vi "Tool Q LEIN stroke fb value ovveride.vi"(1 "Retry on err (F)":bool, 5 "stroke value(mm)":dbl, 9 "Serial number(any number(-1))":i16=-1, 11 "error in (no error)":errorcluster) -> (15 "error out":errorcluster)   [LabVIEW 2011]
doc: "-1 = any address:\n-2 = do not update"
uses:
  LEINmaster/Defenitions/LEIN Structure variations.ctl
  Application Structure/Options/Action GFV Settings.ctl
panel:
  # "-1 = any address:\n-2 =  do not update"
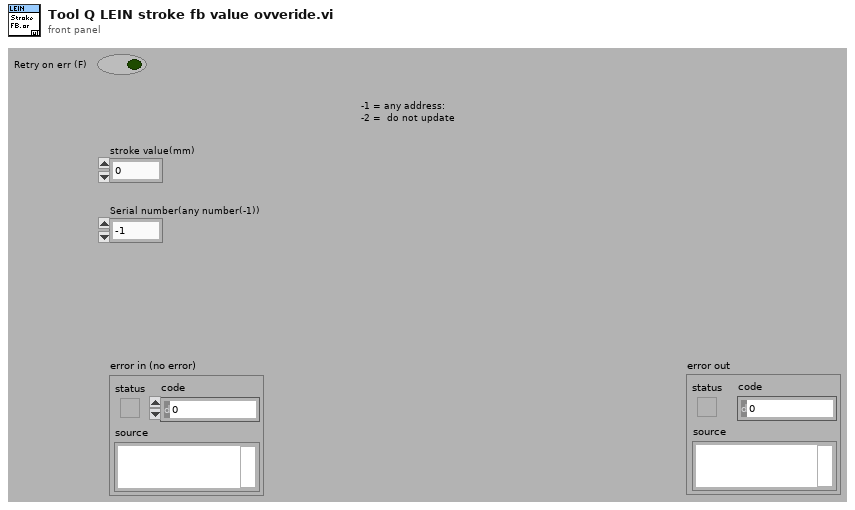
[diagram p1: front panel]
types:
  T1 = typedef "Action GFV Settings.ctl" = enum16{"Init", "Get From INI", "Put In INI", "Get Settings", "Get Update Index", "Set Setting"}
  T2 = typedef "LEIN Structure variations.ctl" = enum16{"LEIN08", "LEIN31", "LEIN63"}
  T3 = enum16{"big-endian, network order", "native, host order", "little-endian"}
  T4 = typedef "Options  All pages and custom.ctl" = cluster{"P 1 (App)":T5, "P 2":T6, "P 3":T7, "P 4":T10, "P 5":T15, "P 6 (Err)":T16, "P 7 (Expert)":T17, "P 8 (Depth)":T19, "C 1":T20, "C 2":T21}
  T5 = typedef "Options Page 1 (App).ctl" = cluster{"Result files":path, "PCP Interface":string, "Tractor/Stroker Interface":string, "Tractor Interface":string, "Modem Status Interface":string, "Audible Alarm":bool, "Force alarm on Technical":bool, "Force alarm on HH":bool, "Force alarm on LL":bool, "Force alarm on H":bool, "Force alarm on L":bool}
  T6 = typedef "Options Page 2.ctl" = cluster{"Solenoid & Relay latching time":u16, "Tractor relay 1":dbl, "Tractor relay 2":dbl, "Tractor Solenoid limit":dbl}
  T7 = typedef "Options Page 3.ctl" = cluster{"Min resistance":dbl, "Max resistance":dbl, "Head voltage range":T8, "Max voltage jump":dbl, "Maximum resistance change":dbl, "Start Telemetry Voltage":dbl, "Start Telemetry Timeout":dbl, "Start Motor Voltage":dbl, "Stop Motor Voltage":dbl, "Pass Mode Warning Voltage":dbl, "Relay Switch Voltage":dbl, "Relay Status Loss Voltage":dbl, "Samples to average":i32, "PSU type DO NOT USE":T9, "Magna OVP":dbl, "Magna Current Limit":dbl}
  T8 = typedef "PCP type List.ctl" = enum16{"0 - 350V", "0 - 450V", "0 - 600V"}
  T9 = typedef "PSU Type.ctl" = enum16{"Unipower", "Magna 8.3A", "Magna 12A", "None"}
  T10 = typedef "Options Page 4.ctl" = cluster{"Solenoid & Relay latching time":u16, "Stroker relay 1":dbl, "Stroker Relay 2":dbl, "Stroker Solenoid limit":dbl, "Force det.":T11, "Stroke force lim.":dbl, "Anchor Enabled Pressure":dbl, "Tacometer puls":dbl, "Default anchor behavior":T12, "Default stroker behavior":T13, "Default stroker force limit (tonne)":dbl, "Slips Size":T14}
  T11 = typedef "Stroke force selector.ctl" = enum16{"Stroke in = node 1", "Strok out = node 1"}
  T12 = typedef "Default anchor behavior.ctl" = enum16{"Do nothing", "Set Anchor", "Release Anchor"}
  T13 = typedef "Default stroker behavior.ctl" = enum16{"Do nothing", "Stop", "Go Out", "Go In"}
  T14 = typedef "Slips Type Radio.ctl" = enum32{"No Selection", "338 MRS", "3,9 MRS"}
  T15 = typedef "Options Page 5.ctl" = cluster{"Solenoid & Relay latching time":u16, "Driller relay 1":dbl, "Driller Relay 2":dbl, "Driller  Solenoid limit":dbl}
  T16 = typedef "Options Page 6 (Err).ctl" = cluster{"Error and event files":path}
  T17 = typedef "Options Page 7 (Expert).ctl" = cluster{"Show Debug":bool, "Log debug messages":bool, "Additional debug messages":bool, "Start Beagle with Simulator data":bool, "Workshop mode":bool, "Modem baud":u16, "enumCANCOM":bool, "Modem sim":T18, "Telemetry Timeout Disable":i32, "Buffer size":i32, "Upd regular data":bool, "Cable comp":cluster{"VMOD1 Voltage(V)":dbl, "VMOD2 Voltage(V)":dbl}}
  T18 = typedef "Modem simulation setup.ctl" = cluster{"Modem dealay sim":bool, "Sim baud Tx":u16, "Bit Error fraction Tx":dbl, "Sim baud Rx":u16, "Bit Error fraction Rx":dbl}
  T19 = typedef "Options Page 8 (Depth).ctl" = cluster{"Winch Spool Circumference":dbl, "Winch Pulses per Revolution":dbl, "Current Depth":dbl}
  T20 = typedef "Options Custom 1.ctl" = cluster{"Depth Updated":bool, "Depth Offset":dbl}
  T21 = typedef "Options Custom 2.ctl" = cluster{"Placeholder":bool}
  T22 = typedef "LEIN CMD Cluster.ctl" = cluster{"SID":u8, "ANF":bool, "CMD":T23, "DATA":u8[]}
  T23 = typedef "LEIN CMD List.ctl" = enum8{"ACTI", "TASK", "RES0", "STAT", "RES1", "RES2", "RES3", "USER"}
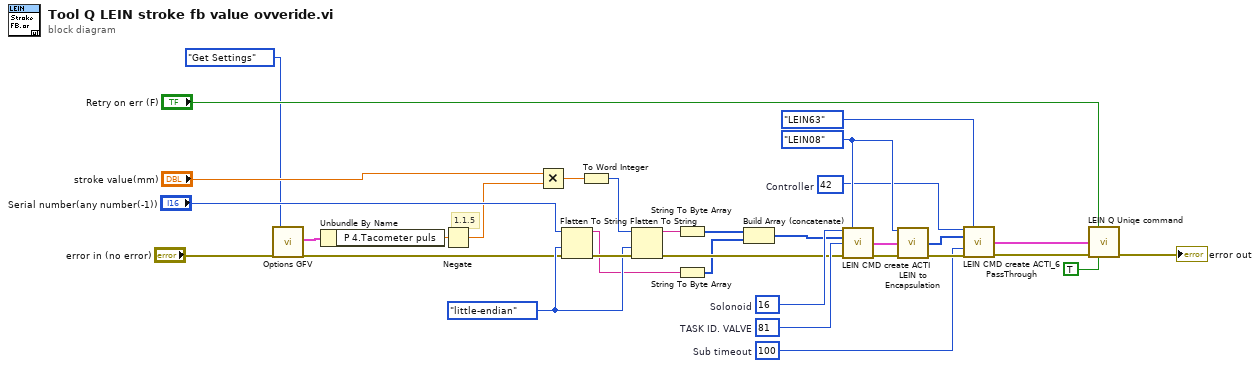
[diagram p0: block diagram]
diagram:
  w16 = u8 42  # Controller
  w17 = u8 16  # Solonoid
  w23 = u16 100  # Sub timeout
  w20 = u8 81  # TASK ID. VALVE
  w19 = LEIN_Structure_variations."LEIN08" ("LEIN Variation")
  w10 = T3."little-endian" ("byte order (0:big-endian, network order)")
  # "1.1.5"
  n1 = call "Options GFV.vi"("error in (no error)"="error in (no error)", "Action(Get Settings)"=Action_GFV_Settings."Get Settings") -> ("Options"=w3:T4, "error out"=w4:errorcluster)  [unwired: 15 in, 1 out]
  n2 = Unbundle By Name(w3) -> ("P 4.Tacometer puls"=w2:dbl)
  n3 = Negate(x=w2) -> (-x=w1:dbl)
  n4 = Multiply(x="stroke value(mm)", y=w1) -> (x*y=w32:dbl)
  n5 = Flatten To String(anything="Serial number(any number(-1))", byte order (0:big-endian, network order)=w10, error in (no error)=w4) -> (data string=w8:string, error out=w11:errorcluster)  [unwired: 1 in, 1 out]
  n6 = To Word Integer(number=w32) -> (16bit integer=w31:i16)
  n7 = Flatten To String(anything=w31, byte order (0:big-endian, network order)=w10, error in (no error)=w11) -> (data string=w30:string, error out=w13:errorcluster)  [unwired: 1 in, 1 out]
  n8 = String To Byte Array(string=w30) -> (unsigned byte array=w18:u8[])
  n9 = String To Byte Array(string=w8) -> (unsigned byte array=w7:u8[])
  n10 = Build Array (concatenate)(w18, w7) -> (w12:u8[])
  n11 = call "LEIN CMD create ACTI.vi"("SID"=w17, "LEIN Variation"=w19, "Data"=w12, "ACTI ID"=w20, "error in (no error)"=w13) -> ("CMD"=w21:T22, "error out"=w22:errorcluster)  [unwired: 9 in]
  n12 = call "LEIN to Encapsulation.vi"("LEIN Variation"=w19, "CMD"=w21, "error in (no error)"=w22) -> ("Data and header"=w26:u8[], "error out"=w27:errorcluster)  [unwired: 8 in, 3 out]
  n13 = call "LEIN CMD create ACTI_6 PassThrough.vi"("SID"=w16, "LEIN Variation"=LEIN_Structure_variations."LEIN63", "LEIN ecapsulated data (header and data)"=w26, "Sub Timeout (ms)"=w23, "error in (no error)"=w27) -> ("CMD"=w25:T22, "error out"=w24:errorcluster)  [unwired: 9 in]
  n14 = call "LEIN Q Uniqe command.vi"("Retry on err (F)"="Retry on err (F)", "CMD"=w25, "error in"=w24, "priority(F)"=TRUE) -> ("error out"=→"error out":errorcluster)  [unwired: 11 in]
